vi "Drivetrain Past Target.vi"(6 "Use X Distance?":bool, 8 "Forward Only?":bool, 9 "Distance Target":dbl, 11 "Reset":bool) -> (3 "Past Target?":bool)   [LabVIEW 2014]
uses:
  Robot Global Data.vi
panel:
  out "Start Dist":dbl
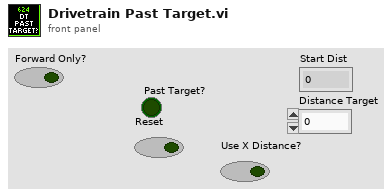
[diagram p1: front panel]
types:
  T1 = typedef "Encoder Values.ctl" = cluster{"Distance":dbl, "Speed":dbl, "Ticks":dbl}
  T2 = cluster{"Left Encoder":T1, "Center Encoder":T1, "Right Encoder":T1}
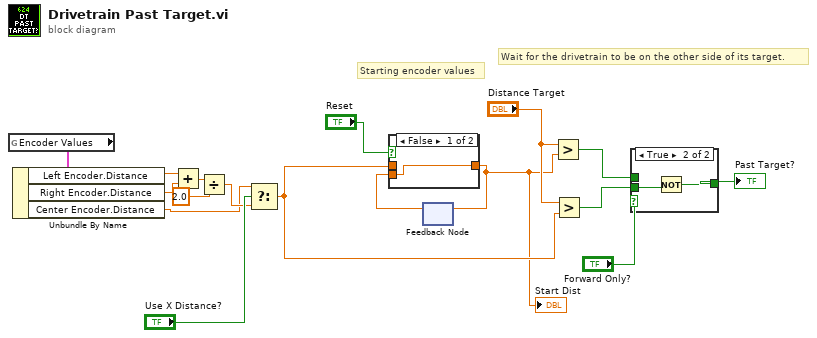
[diagram p0: block diagram]
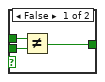
[diagram p2: hidden frame]
diagram:
  # "Wait for the drivetrain to be on the other side of its target."
  # "Starting encoder values"
  n1 = global read "Robot Global Data.vi" "Encoder Values"() -> (w17:T2)
  n2 = Unbundle By Name(w17) -> ("Left Encoder.Distance"=w16:dbl, "Right Encoder.Distance"=w15:dbl, "Center Encoder.Distance"=w6:dbl)
  n3 = Add(x=w16, y=w15) -> (x+y=w14:dbl)
  n4 = Divide(x=w14, y=2.0) -> (x/y=w7:dbl)
  n5 = Select(t=w6, s="Use X Distance?", f=w7) -> (s? t:f=w4:dbl)
  n6 = feedback #1() -> (w12:dbl)  [unwired: 1 in]
  n7 = case shown="False" "Reset" {
    tunnel: [w18 w19] -> w3
    tunnel: w12 -> [w18 _]
    tunnel: w4 -> [_ w19]
    frame False {
    }
    frame True {
    }
  }
  "Start Dist" <- w3
  n8 = feedback-in #1(w3) -> ()
  n9 = Greater?(x="Distance Target", y=w3) -> (0:w10:bool)
  n10 = Greater?(x="Distance Target", y=w4) -> (0:w2:bool)
  n11 = case shown="True" "Forward Only?" {
    tunnel: w10 -> [w22 _]
    tunnel: w2 -> [w21 w24]
    tunnel: [w20 w23] -> w5
    frame False {
      n12 = Not Equal?(x=w22, y=w21) -> (x != y?=w20:bool)
    }
    frame True {
      n13 = Not(x=w24) -> (.not. x?=w23:bool)
    }
  }
  "Past Target?" <- w5
